vi "wait on clock.vi"(8 "error in":errorcluster, 10 "dt":u32=1, 11 "timing source in":refnum<class "ms timing source.lvclass">) -> (0 "error out":errorcluster, 2 "ticks since last call":u32, 3 "timing source out":refnum<class "ms timing source.lvclass">)   [LabVIEW 2013, in "ms timing source.lvclass"]
doc: "This core timing function is used inside of a loop to wait for a clock signal, or dt ticks of a clock signal."
uses:
  ms timing source.lvclass
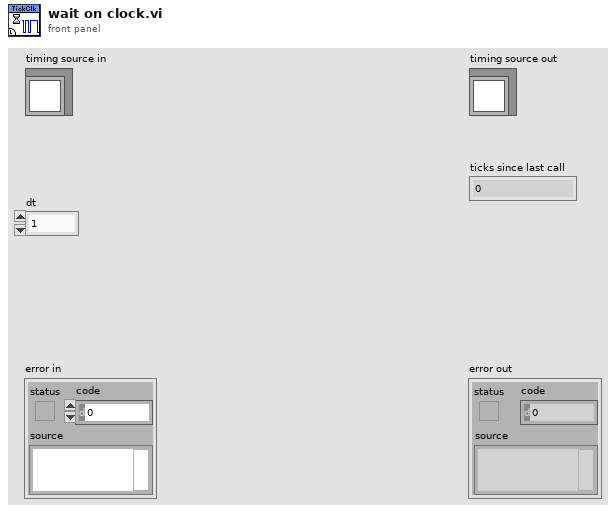
[diagram p1: front panel]
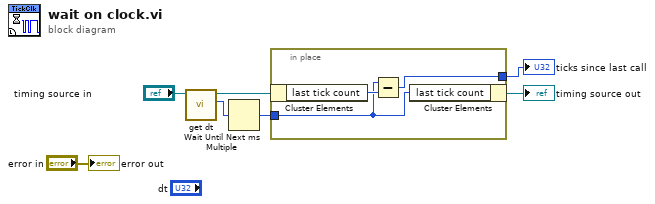
[diagram p0: block diagram]
diagram:
  n1 = call "get dt.vi"("timing source in"="timing source in") -> ("dt"=w2:u32, "timing source out"=w5:refnum<class "ms timing source.lvclass">)  [unwired: 9 in]
  n2 = Wait Until Next ms Multiple(millisecond multiple=w2) -> (millisecond timer value=w1:u32)
  n3 = in-place {
    in-place-border: [w9] -> w3
    in-place-border: w1 -> [w8]
    n4 = in-place-cluster #1(w5) -> ("last tick count"=w10:u32)
    n5 = Subtract(x=w8, y=w10) -> (x-y=w9:u32)
    n6 = in-place-cluster #1("last tick count"=w8) -> (→"timing source out":refnum<class "ms timing source.lvclass">)
  }
  "ticks since last call" <- w3
  "error out" <- "error in"
